vi "user prompt face problem.vi"(0 "Enable":bool=TRUE, 5 "error in (no error)":errorcluster) -> (18 "OK":bool, 19 "error out":errorcluster)   [LabVIEW 2019]
doc: "Displays a standard dialog box that prompts users to enter information, such as a user name and password.\n--------------------\n\nThis Express VI is configured as follows:\n\nMessage to Display to the User:\nThe inputs are:"
panel:
  out "?":u32(colorbox)
  in  "?":u32(colorbox)
  out "?":u32(colorbox)
  out "?":u32(colorbox)
  out "?":u32(colorbox)
  out "?":u32(colorbox)
  out "?":u32(colorbox)
  out "?":u32(colorbox)
  out "?":u32(colorbox)
  out "?":u32(colorbox)
  out "?":u32(colorbox)
  out "?":u32(colorbox)
  out "?":u32(colorbox)
  out "?":u32(colorbox)
  out "?":u32(colorbox)
  out "?":u32(colorbox)
  out "?":u32(colorbox)
  out "?":u32(colorbox)
  out "?":u32(colorbox)
  out "?":u32(colorbox)
  out "?":u32(colorbox)
  out "?":u32(colorbox)
  out "?":u32(colorbox)
  out "?":u32(colorbox)
  out "?":u32(colorbox)
  out "?":u32(colorbox)
  out "?":u32(colorbox)
  out "?":u32(colorbox)
  out "?":u32(colorbox)
  out "?":u32(colorbox)
  out "?":u32(colorbox)
  out "?":u32(colorbox)
  out "?":u32(colorbox)
  out "?":u32(colorbox)
  out "?":u32(colorbox)
  out "?":u32(colorbox)
  out "?":u32(colorbox)
  out "?":u32(colorbox)
  out "?":u32(colorbox)
  out "?":u32(colorbox)
  out "?":u32(colorbox)
  out "?":u32(colorbox)
  out "?":u32(colorbox)
  out "?":u32(colorbox)
  out "?":u32(colorbox)
  out "?":u32(colorbox)
  out "?":u32(colorbox)
  out "?":u32(colorbox)
  out "?":u32(colorbox)
  out "?":u32(colorbox)
  out "?":u32(colorbox)
  out "?":u32(colorbox)
  out "?":u32(colorbox)
  out "?":u32(colorbox)
  out "?":u32(colorbox)
  out "?":u32(colorbox)
  out "String":string
  in  "Cancel":bool
  in  "OK2":bool
  in  "OK1":bool
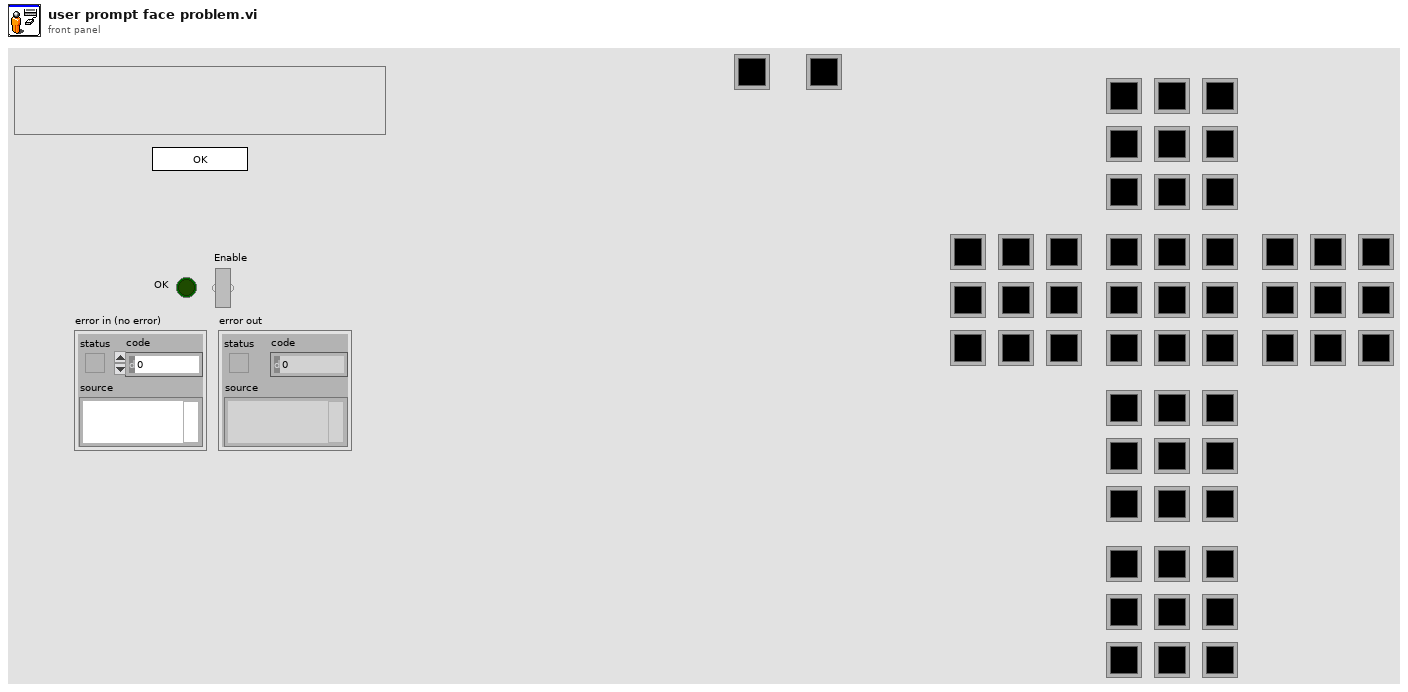
[diagram p1: front panel]
types:
  T1 = cluster{"Input Name":string, "Input Data Type":i32}[]
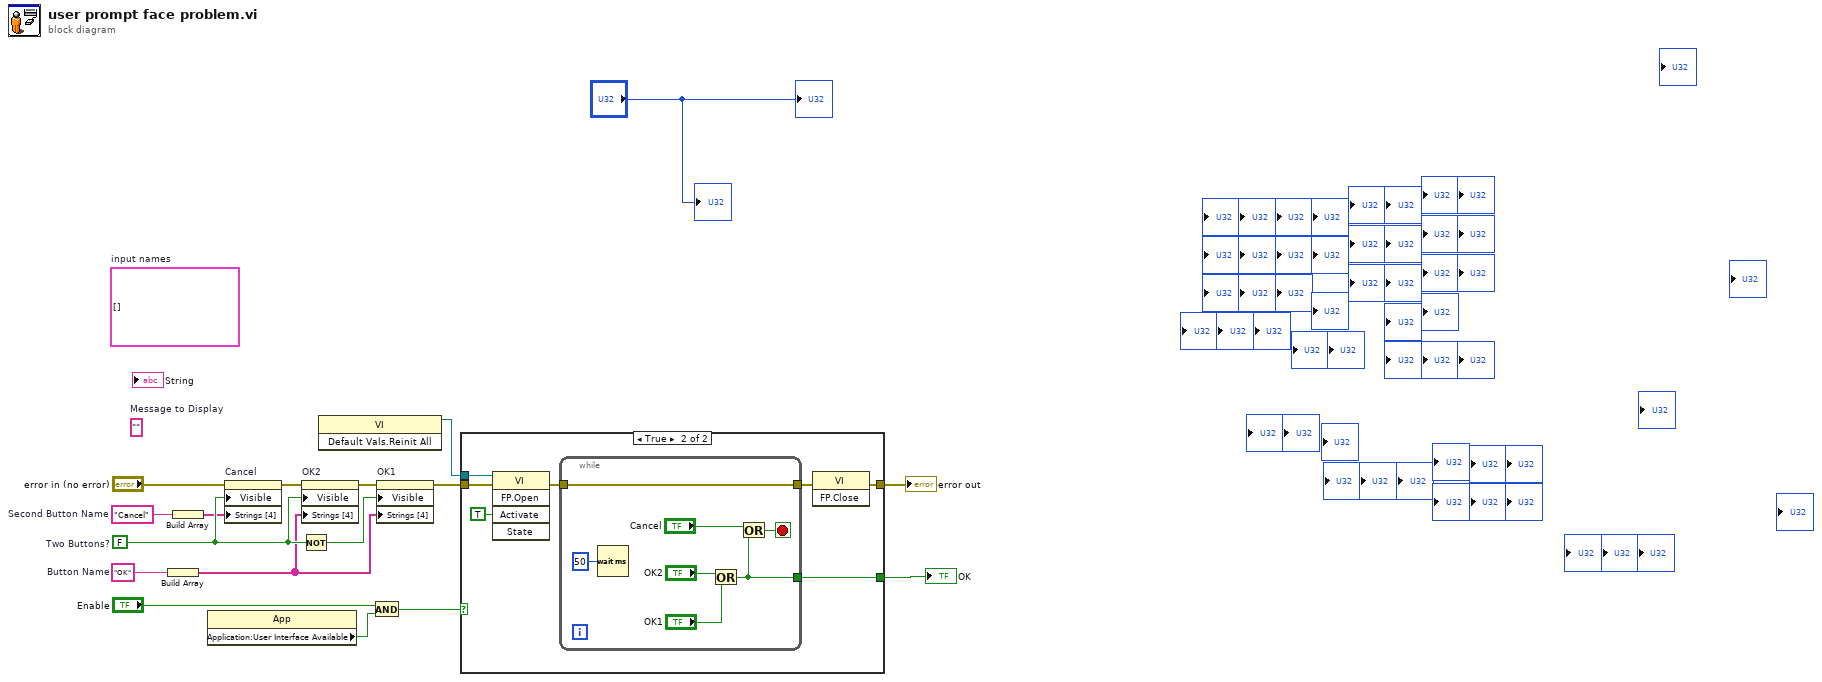
[diagram p0: block diagram]
diagram:
  (unwired) T1 []  # input names
  w11 = "Cancel"  # Second Button Name
  w9 = "OK"  # Button Name
  (unwired) ""  # Message to Display
  w17 = FALSE  # Two Buttons?
  n1 = Build Array(w9) -> (w10:string[])
  n2 = Build Array(w11) -> (w12:string[])
  n3 = property class="App"() -> ("Application:User Interface Available"=w4:bool)  [unwired: 2 in, 2 out]
  n4 = property on="Cancel" class="Bool"(error in="error in (no error)", "Visible"=w17, "Strings [4]"=w12) -> (error out=w14:errorcluster)  [unwired: 1 in, 1 out]
  n5 = Not(x=w17) -> (.not. x?=w15:bool)
  n6 = property on="OK2" class="Bool"(error in=w14, "Visible"=w17, "Strings [4]"=w10) -> (error out=w13:errorcluster)  [unwired: 1 in, 1 out]
  n7 = invoke class="VI" method="Default Vals.Reinit All"() -> (reference out=w3:refnum<vi>)  [unwired: 3 in, 2 out]
  n8 = And(x="Enable", y=w4) -> (x .and. y?=w2:bool)
  n9 = property on="OK1" class="Bool"(error in=w13, "Visible"=w15, "Strings [4]"=w10) -> (error out=w8:errorcluster)  [unwired: 1 in, 1 out]
  n10 = case shown="True" w2 {
    tunnel: [_ w25] -> w16
    tunnel: w8 -> [w18 w24]
    tunnel: [w18 w23] -> w6
    tunnel: w3 -> [_ w22]
    frame False {
    }
    frame True {
      n11 = invoke class="VI" method="FP.Open"(reference=w22, error in=w24, "Activate"=TRUE ("Activate?")) -> (error out=w20:errorcluster)  [unwired: 2 in, 4 out]
      n12 = while "Main While Loop" {
        tunnel: [w29] -> w25
        tunnel: w20 -> [w26]
        tunnel: [w26] -> w19
        stop <- w27 stop-if-true
        n13 = Wait (ms)(milliseconds to wait=u32 50 ("millisecond multiple")) -> ()  [unwired: 1 out]
        n14 = Or(x="OK2", y="OK1") -> (x .or. y?=w29:bool)
        n15 = Or(x="Cancel", y=w29) -> (x .or. y?=w27:bool)
      }
      n16 = invoke class="VI" method="FP.Close"(error in=w19) -> (error out=w23:errorcluster)  [unwired: 2 in, 2 out]
    }
  }
  "OK" <- w16
  "error out" <- w6
  "?" <- "?"
  "?" <- "?"
